vi "d Hi--C1.vi"(8 "Command Info In":T2, 10 "d Hi--C1":T1={"1a"=38.0, "1d"=18.0, "1s"=0.75, "3t"=0.0, "4d"=0.0, "4s"=0.0}, 11 "Scale":string) -> (0 "Command Info Out":T2)   [LabVIEW 2017]
uses:
  <vilib>/Rock Robotics/WPI/Framework/Command Status Info.ctl
  <vilib>/Rock Robotics/WPI/Framework/Completion Status.ctl
  <vilib>/Rock Robotics/WPI/Framework/Completion Notifier.ctl
  Block Clusters/d Hi--C1.ctl
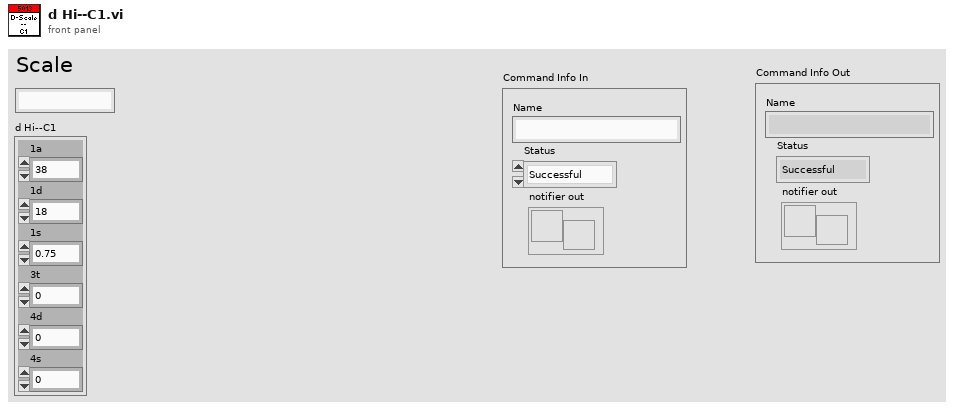
[diagram p1: front panel]
types:
  T1 = typedef "d Hi--C1.ctl" = cluster{"1a":dbl, "1d":dbl, "1s":dbl, "3t":dbl, "4d":dbl, "4s":dbl}
  T2 = typedef "Command Status Info.ctl" = cluster{"Name":string, "Status":T3, "notifier out":T4}
  T3 = typedef "Completion Status.ctl" = enum16{"Successful", "Aborted", "Incomplete"}
  T4 = typedef "Completion Notifier.ctl" = refnum<notifier>
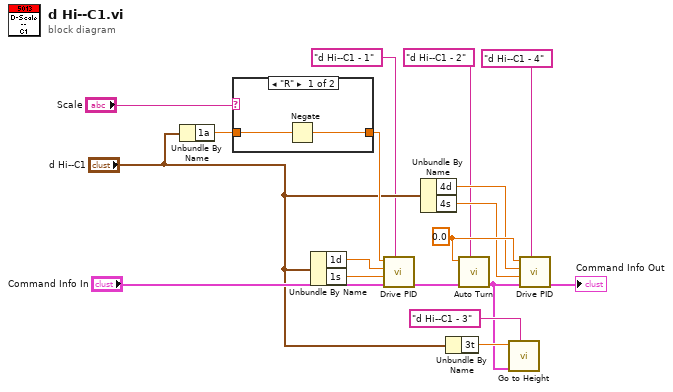
[diagram p0: block diagram]
diagram:
  w8 = 0.0 ("Target Angle")
  n1 = Unbundle By Name("d Hi--C1") -> ("1a"=w18:dbl)
  n2 = case shown="\"R\"" "Scale" {
    tunnel: w18 -> [w20 w21]
    tunnel: [w19 w21] -> w17
    frame "R" {
      n3 = Negate(x=w20) -> (-x=w19:dbl)
    }
    frame "L", Default {
    }
  }
  n4 = Unbundle By Name("d Hi--C1") -> ("1d"=w15:dbl, "1s"=w16:dbl)
  n5 = call "Drive PID.vi"("Description"="d Hi--C1 - 1", "Command Info In"="Command Info In", "Speed"=w16, "Distance"=w15, "Target Angle"=w17) -> ("Command Info Out"=w11:T2)  [unwired: 6 in]
  n6 = Unbundle By Name("d Hi--C1") -> ("4d"=w7:dbl, "4s"=w6:dbl)
  n7 = Unbundle By Name("d Hi--C1") -> ("3t"=w13:dbl)
  n8 = call "Auto Turn.vi"("Description"="d Hi--C1 - 2", "Command Info In"=w11, "Target Angle"=w8) -> ("Command Info Out"=w2:T2)  [unwired: 8 in]
  n9 = call "Go to Height.vi"("Description"="d Hi--C1 - 3", "Command Info In"=w2, "Target Height (in)"=w13) -> ()  [unwired: 8 in, 1 out]
  n10 = call "Drive PID.vi"("Description"="d Hi--C1 - 4", "Command Info In"=w2, "Speed"=w6, "Distance"=w7, "Target Angle"=w8) -> ("Command Info Out"=→"Command Info Out":T2)  [unwired: 6 in]
